vi "FTW-TestExecutive-Core_Step.vi"(0 "FTW-TestExecutive-Core In":refnum<class "FTW-TestExecutive-Core.lvclass">, 11 "error in":errorcluster) -> (4 "FTW-TestExecutive-Core Out":refnum<class "FTW-TestExecutive-Core.lvclass">, 15 "error out":errorcluster)   [LabVIEW 2015, in "FTW-TestExecutive-Core.lvclass"]
uses:
  FTW-TestExecutive-Core.lvclass
  FTW-TestExecutive-Core.lvclass/FTW-TestExecutive-Core.ctl
  FTW-TestExecutive-Core_State.ctl
  Instance/FTW-ActorInstance.lvclass
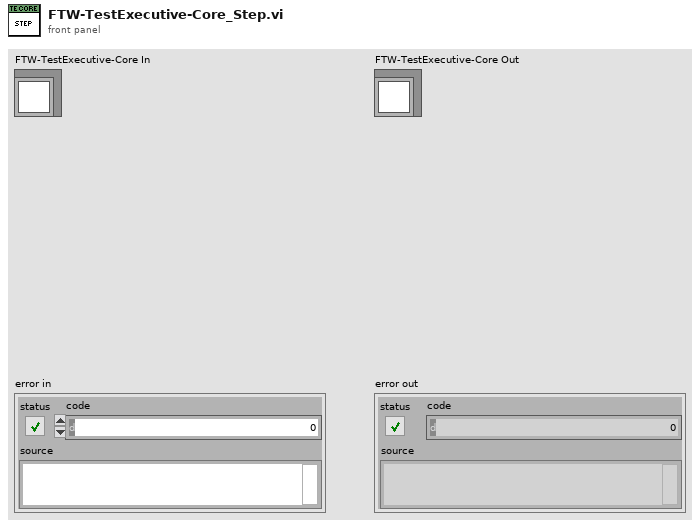
[diagram p1: front panel]
types:
  T1 = typedef "FTW-TestExecutive-Core.lvclass/FTW-TestExecutive-Core_State.ctl" = enum8{"Unloaded", "Loaded", "Executing", "Paused"}
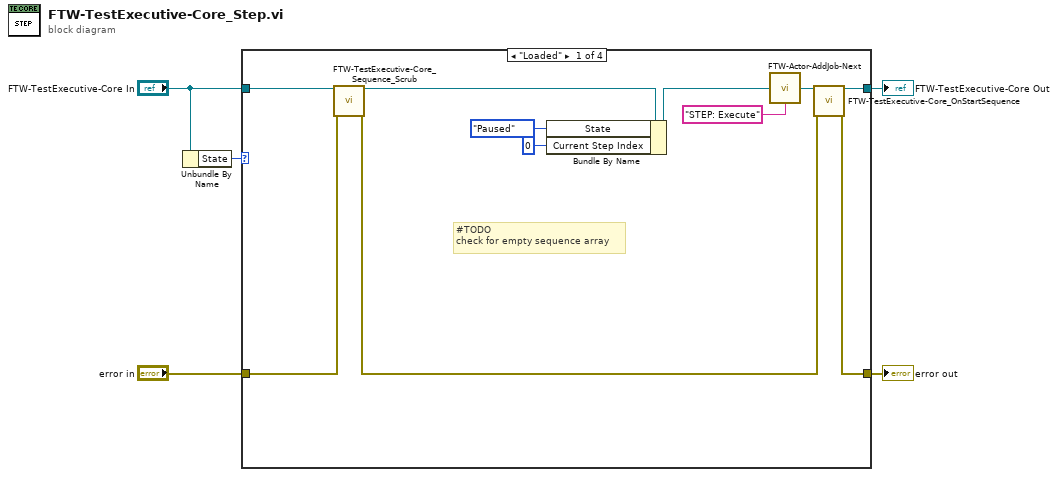
[diagram p0: block diagram]
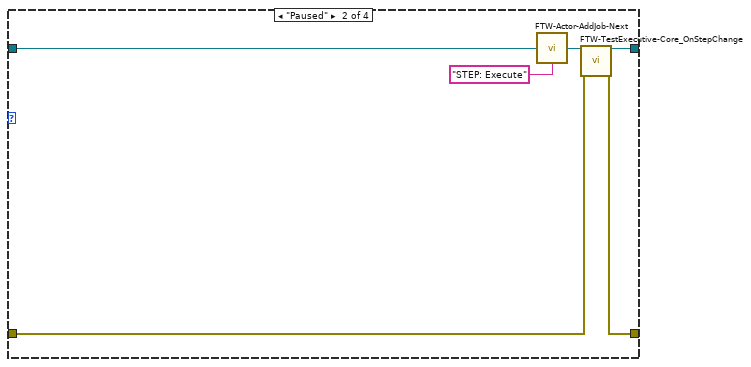
[diagram p2: hidden frame]
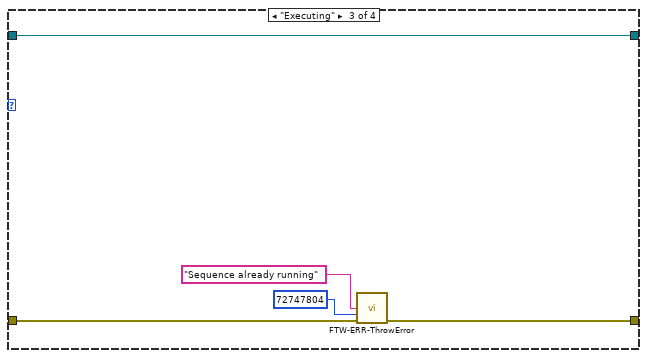
[diagram p3: hidden frame]
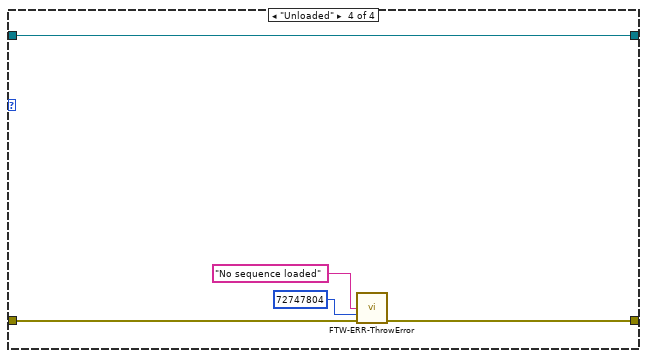
[diagram p4: hidden frame]
diagram:
  n1 = Unbundle By Name("FTW-TestExecutive-Core In") -> ("State"=w3:T1)
  n2 = case shown="\"Loaded\"" w3 {
    tunnel: [w10 w19 w27 w32] -> w5
    tunnel: "FTW-TestExecutive-Core In" -> [w14 w22 w27 w32]
    tunnel: [w9 w18 w25 w30] -> w2
    tunnel: "error in" -> [w7 w17 w26 w31]
    frame "Loaded" {
      # "#TODO\ncheck for empty sequence array"
      n3 = call "FTW-TestExecutive-Core_Sequence_Scrub.vi"("FTW-TestExecutive-Core In"=w14, "error in"=w7) -> ("FTW-TestExecutive-Core Out"=w8:refnum<class "FTW-TestExecutive-Core.lvclass">, "error out"=w6:errorcluster)  [unwired: 12 in]
      n4 = Bundle By Name(cluster=w8, "State"=FTW-TestExecutive-Core_State."Paused", "Current Step Index"=0 ("Pointer")) -> (w16:refnum<class "FTW-TestExecutive-Core.lvclass">)
      n5 = call "FTW-Actor-AddJob-Next.vi"("Add Next in Job Queue"="STEP: Execute", "FTW Actor Instance"=w16) -> ("FTW Actor Instance out"=w12:refnum<class "FTW-TestExecutive-Core.lvclass">)  [unwired: 2 in]
      n6 = call "FTW-TestExecutive-Core_OnStartSequence.vi"("FTW-TestExecutive-Core In"=w12, "error in"=w6) -> ("FTW-TestExecutive-Core Out"=w10:refnum<class "FTW-TestExecutive-Core.lvclass">, "error out"=w9:errorcluster)  [unwired: 12 in]
    }
    frame "Paused" {
      n7 = call "FTW-Actor-AddJob-Next.vi"("Add Next in Job Queue"="STEP: Execute", "FTW Actor Instance"=w22) -> ("FTW Actor Instance out"=w21:refnum<class "FTW-TestExecutive-Core.lvclass">)  [unwired: 2 in]
      n8 = call "FTW-TestExecutive-Core_OnStepChange.vi"("FTW-TestExecutive-Core In"=w21, "error in"=w17) -> ("FTW-TestExecutive-Core Out"=w19:refnum<class "FTW-TestExecutive-Core.lvclass">, "error out"=w18:errorcluster)  [unwired: 12 in]
    }
    frame "Executing" {
      n9 = call "FTW-ERR-ThrowError.vi"("Error Message"="Sequence already running", "Error Code"=72747804, "error in"=w26) -> ("error out"=w25:errorcluster)  [unwired: 12 in]
    }
    frame "Unloaded" {
      n10 = call "FTW-ERR-ThrowError.vi"("Error Message"="No sequence loaded", "Error Code"=72747804, "error in"=w31) -> ("error out"=w30:errorcluster)  [unwired: 12 in]
    }
  }
  "FTW-TestExecutive-Core Out" <- w5
  "error out" <- w2
